vi "FTW-ActorExtended-Initialize.vi"(0 "FTW Actor Instance Type":refnum<class "FTW-ActorExtended.lvclass">, 5 "Initialization Job Sequence":string, 7 "Actor Instance Configuration":string, 11 "error in":errorcluster) -> (4 "FTW Actor Instance":refnum<class "FTW-ActorExtended.lvclass">, 6 "Event Refnums":T1, 15 "error out":errorcluster)   [LabVIEW 2015, in "FTW-ActorExtended.lvclass"]
uses:
  FTW-ActorExtended.lvclass
  Message/Request/FTW-Message-IncomingRequest.lvclass
  Message/Base/FTW-Message.lvclass
  FTW-ActorExtended.lvclass/FTW-ActorExtended.ctl
  Connector/FTW-ActorConnector.lvclass
  Subscriber/FTW-Subscriber.lvclass
  Publisher/FTW-Publisher.lvclass
panel:
  # "Inputs"
  # "Outputs"
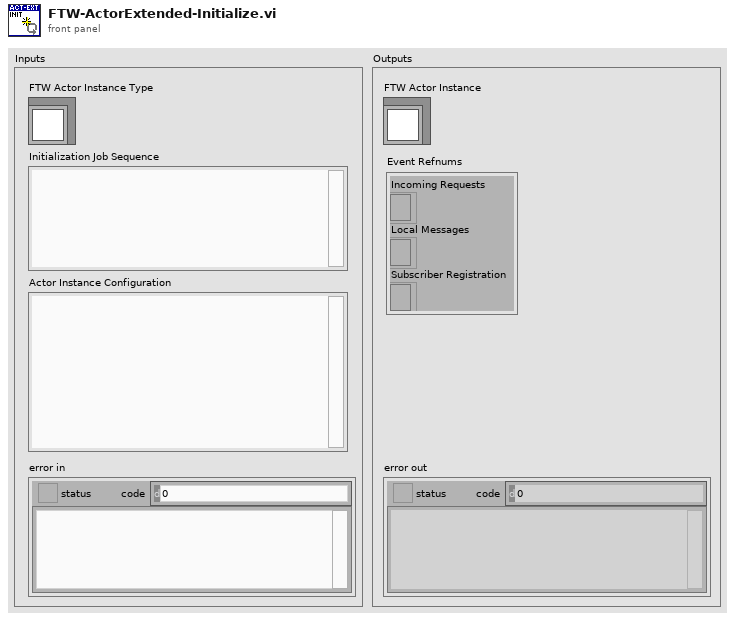
[diagram p1: front panel]
types:
  T1 = cluster{"Incoming Requests":refnum<event-registration>, "Local Messages":refnum<event-registration>, "Subscriber Registration":refnum<event-registration>}
  T2 = cluster{"String":string, "LabVIEW String":string, "FTW Actor Connector":refnum<class "FTW-ActorConnector.lvclass">, bool}
  T3 = cluster{"String":string, "Actual Address":string, "FTW-Publisher Out":refnum<class "FTW-Publisher.lvclass">}
  T4 = typedef "FTW-JSON-Type.ctl" = enum8{"Not Found", "Object", "Array", "String", "Number", "Boolean", "null"}
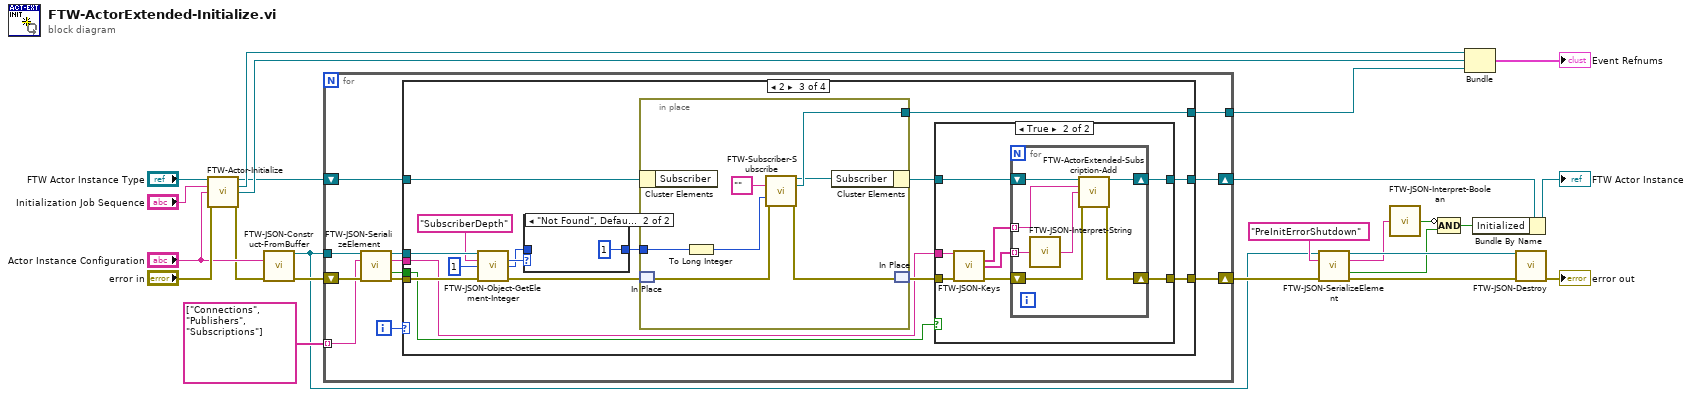
[diagram p0: block diagram]
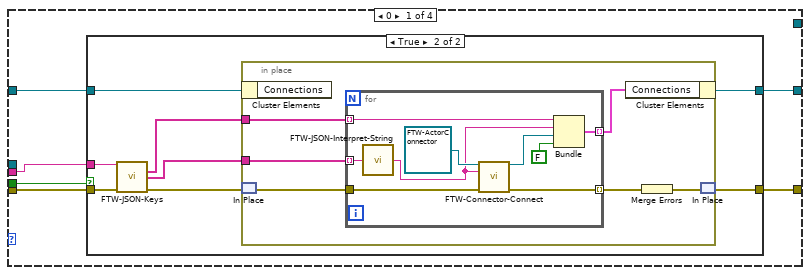
[diagram p2: hidden frame]
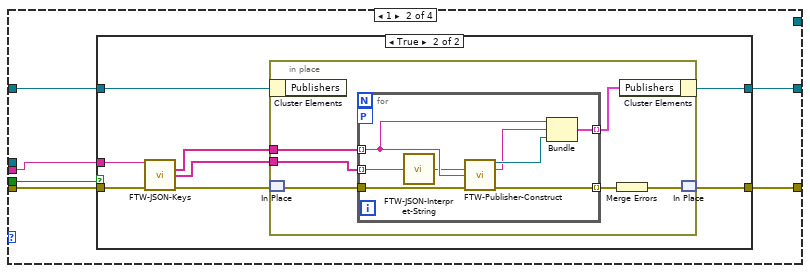
[diagram p4: hidden frame]
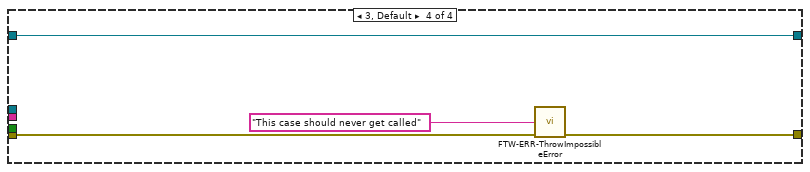
[diagram p8: hidden frame]
diagram:
  n1 = call-dynamic "FTW-Actor-Initialize.vi"("FTW Actor Instance Type"="FTW Actor Instance Type", "Initialization Job Sequence"="Initialization Job Sequence", "Actor Instance Configuration"="Actor Instance Configuration", "error in"="error in") -> ("FTW Actor Instance"=w15:refnum<class "FTW-ActorExtended.lvclass">, "Incoming Requests"=w21:refnum<event-registration>, "Local Messages"=w20:refnum<event-registration>, "error out"=w17:errorcluster)  [unwired: 8 in]
  n2 = call "FTW-JSON-Construct-FromBuffer.vi"("JSON String (UTF-8)"="Actor Instance Configuration", "error in"=w17) -> ("JSON"=w2:refnum<class "FTW-Container.lvclass">, "error out"=w16:errorcluster)  [unwired: 12 in]
  n3 = for {
    tunnel: w2 -> [w36]
    tunnel: string[] ["Connections", "Publishers", "Subscriptions"] -> [w34] mode=indexing
    shift-right: [w29] -> w14
    shift-left: w15 -> [w30]
    shift-right: [w28] -> w13
    shift-left: w16 -> [w35]
    tunnel: [w27] -> w12
    i -> [w33]
    n4 = call "FTW-JSON-SerializeElement.vi"("JSON"=w36, "Key"=w34, "error in"=w35) -> ("JSON out"=w26:refnum<class "FTW-Container.lvclass">, "Element as JSON String"=w32:string, "Found?"=w25:bool, "error out"=w31:errorcluster)  [unwired: 9 in]
    n5 = case shown="2" w33 {
      tunnel: w32 -> [w38 w69 w109 _]
      tunnel: w31 -> [w40 w71 w112 w142]
      tunnel: w30 -> [w42 w73 w113 w143]
      tunnel: [w41 w72 w106 w143] -> w29
      tunnel: [w39 w70 w108 w141] -> w28
      tunnel: [_ _ w110 _] -> w27
      tunnel: w26 -> [_ _ w104 _]
      tunnel: w25 -> [w37 w68 w99 _]
      frame 0 {
        n6 = case shown="True" w37 {
          tunnel: w42 -> [w44 w52]
          tunnel: [w44 w51] -> w41
          tunnel: w40 -> [w43 w50]
          tunnel: [w43 w46] -> w39
          tunnel: w38 -> [_ w45]
          frame False {
          }
          frame True {
            n7 = call "FTW-JSON-Keys.vi"("JSON Opject"=w45, "error in"=w50) -> ("Keys"=w49:string[], "Values"=w48:string[], "error out"=w47:errorcluster)  [unwired: 11 in]
            n8 = in-place {
              in-place-border: w49 -> [w54]
              in-place-border: w48 -> [w58]
              n9 = in-place-cluster #1(w52) -> ()  [unwired: 1 out]
              n10 = in-place-match #2(w47) -> (w56:errorcluster)
              n11 = for {
                tunnel: w56 -> [w65]
                tunnel: w58 -> [w66] mode=indexing
                tunnel: [w67] -> w57 mode=indexing
                tunnel: w54 -> [w63] mode=indexing
                tunnel: [w60] -> w53 mode=indexing
                n12 = call "FTW-JSON-Interpret-String.vi"("JSON String"=w66) -> ("LabVIEW String"=w62:string)
                n13 = call-dynamic "FTW-Connector-Connect.vi"("FTW Actor Connector Type"=refnum<class "FTW-ActorConnector.lvclass"> refnum, "Instance Inbox Address"=w62, "error in"=w65) -> ("FTW Actor Connector"=w61:refnum<class "FTW-ActorConnector.lvclass">, "error out"=w67:errorcluster)  [unwired: 11 in]
                n14 = Bundle("String"=w63, "LabVIEW String"=w62, "FTW Actor Connector"=w61, FALSE) -> (w60:T2)  [unwired: 1 in]
              }
              n15 = in-place-cluster #1("Connections"=w53) -> (w51:refnum<class "FTW-ActorExtended.lvclass">)
              n16 = Merge Errors(w57) -> (w55:errorcluster)
              n17 = in-place-match #2(w55) -> (w46:errorcluster)
            }
          }
        }
      }
      frame 1 {
        n18 = case shown="True" w68 {
          tunnel: w73 -> [w75 w83]
          tunnel: [w75 w82] -> w72
          tunnel: w71 -> [w74 w81]
          tunnel: [w74 w77] -> w70
          tunnel: w69 -> [_ w76]
          frame False {
          }
          frame True {
            n19 = call "FTW-JSON-Keys.vi"("JSON Opject"=w76, "error in"=w81) -> ("Keys"=w80:string[], "Values"=w79:string[], "error out"=w78:errorcluster)  [unwired: 11 in]
            n20 = in-place {
              in-place-border: w80 -> [w84]
              in-place-border: w79 -> [w89]
              n21 = in-place-cluster #3(w83) -> ()  [unwired: 1 out]
              n22 = in-place-match #4(w78) -> (w87:errorcluster)
              n23 = for {
                tunnel: w87 -> [w96]
                tunnel: w89 -> [w97] mode=indexing
                tunnel: w84 -> [w94] mode=indexing
                tunnel: [w95] -> w88 mode=indexing
                workers-P: _ -> [_]
                tunnel: [w90] -> w85 mode=indexing
                n24 = call "FTW-JSON-Interpret-String.vi"("JSON String"=w97) -> ("LabVIEW String"=w93:string)
                n25 = call "FTW-Publisher-Construct.vi"("Address"=w93, "Identity"=w94, "error in"=w96) -> ("FTW-Publisher Out"=w92:refnum<class "FTW-Publisher.lvclass">, "Actual Address"=w91:string, "error out"=w95:errorcluster)  [unwired: 10 in]
                n26 = Bundle("String"=w94, "Actual Address"=w91, "FTW-Publisher Out"=w92) -> (w90:T3)  [unwired: 1 in]
              }
              n27 = Merge Errors(w88) -> (w86:errorcluster)
              n28 = in-place-cluster #3("Publishers"=w85) -> (w82:refnum<class "FTW-ActorExtended.lvclass">)
              n29 = in-place-match #4(w86) -> (w77:errorcluster)
            }
          }
        }
      }
      frame 2 {
        n30 = call "FTW-JSON-Object-GetElement-Integer.vi"("JSON"=w104, "Key"="SubscriberDepth", "Default Value"=i64 1, "error in"=w112) -> ("JSON Element Type"=w102:T4, "Value"=w100:i64, "error out"=w105:errorcluster)  [unwired: 8 in, 1 out]
        n31 = case shown="\"Not Found\", Default" w102 {
          tunnel: [w131 i64 1 ("f")] -> w101
          tunnel: w100 -> [w131 _]
          frame "Number" {
          }
          frame "Not Found", Default {
          }
        }
        n32 = in-place {
          in-place-border: [w137] -> w110
          in-place-border: w101 -> [w134]
          n33 = in-place-cluster #5(w113) -> ()  [unwired: 1 out]
          n34 = in-place-match #6(w105) -> (w139:errorcluster)
          n35 = To Long Integer(number=w134) -> (32bit integer=w133:i32)
          n36 = call "FTW-Subscriber-Subscribe.vi"("Addresses"="" ("empty string"), "Buffer Depth (1 element)"=w133, "error in"=w139) -> ("FTW-Subscription Out"=w135:refnum<class "FTW-Subscriber.lvclass">, "Subscriber Registration"=w137:refnum<event-registration>, "error out"=w138:errorcluster)  [unwired: 10 in]
          n37 = in-place-cluster #5("Subscriber"=w135) -> (w107:refnum<class "FTW-ActorExtended.lvclass">)
          n38 = in-place-match #6(w138) -> (w111:errorcluster)
        }
        n39 = case shown="True" w99 {
          tunnel: w111 -> [w114 w123]
          tunnel: w109 -> [_ w121]
          tunnel: [w114 w120] -> w108
          tunnel: w107 -> [w115 w119]
          tunnel: [w115 w118] -> w106
          frame False {
          }
          frame True {
            n40 = call "FTW-JSON-Keys.vi"("JSON Opject"=w121, "error in"=w123) -> ("Keys"=w116:string[], "Values"=w117:string[], "error out"=w122:errorcluster)  [unwired: 11 in]
            n41 = for {
              shift-right: [w127] -> w118
              shift-left: w119 -> [w128]
              shift-right: [w129] -> w120
              shift-left: w122 -> [w130]
              tunnel: w117 -> [w126] mode=indexing
              tunnel: w116 -> [w124] mode=indexing
              n42 = call "FTW-JSON-Interpret-String.vi"("JSON String"=w126) -> ("LabVIEW String"=w125:string)
              n43 = call "FTW-ActorExtended-Subscription-Add.vi"("FTW-ActorExtended In"=w128, "Subscriber Name"=w124, "Subscriber URI"=w125, "error in"=w130) -> ("FTW-ActorExtended Out"=w127:refnum<class "FTW-ActorExtended.lvclass">, "error out"=w129:errorcluster)  [unwired: 10 in]
            }
          }
        }
      }
      frame 3, Default {
        n44 = call "FTW-ERR-ThrowImpossibleError.vi"("Reason this error should never happen"="This case should never get called", "error in"=w142) -> ("error out"=w141:errorcluster)  [unwired: 13 in]
      }
    }
  }
  n45 = call "FTW-JSON-SerializeElement.vi"("JSON"=w2, "Key"="PreInitErrorShutdown", "error in"=w13) -> ("JSON out"=w7:refnum<class "FTW-Container.lvclass">, "Element as JSON String"=w5:string, "Found?"=w1:bool, "error out"=w8:errorcluster)  [unwired: 9 in]
  n46 = call "FTW-JSON-Interpret-Boolean.vi"("JSON Boolean"=w5) -> ("LabVIEW Boolean"=w4:bool)
  n47 = Compound Arithmetic op=AND(invert w4, w1) -> (w3:bool)
  n48 = Bundle("Incoming Requests"=w21, "Local Messages"=w20, "Subscriber Registration"=w12) -> (→"Event Refnums":T1)  [unwired: 1 in]
  n49 = Bundle By Name(cluster=w14, "Initialized"=w3) -> (→"FTW Actor Instance":refnum<class "FTW-ActorExtended.lvclass">)
  n50 = call "FTW-JSON-Destroy.vi"("JSON"=w7, "error in"=w8) -> ("error out"=→"error out":errorcluster)  [unwired: 13 in]
